vi "Begin.vi"(8 "error in":errorcluster) -> (0 "error out":errorcluster)   [LabVIEW 2023]
doc: "Called before other user functions, this VI is expected to open initial I/O refnums, load in file data, and do all program initialization. Notice that the <B>error out</B> terminal is simply used for data flow. Wiring it to other structures or subVIs ensures that this VI runs first."
uses:
  <vilib>/Rock Robotics/WPI/DriverStation/WPI_DriverStationRobotMode2.ctl
  Robot Global Data.vi
  <vilib>/Rock Robotics/Network Tables/NT Write String Array.vi
  <vilib>/Rock Robotics/WPI/ThirdParty/JAS_Junk/TrajLib/Trajectory_Library.lvlib
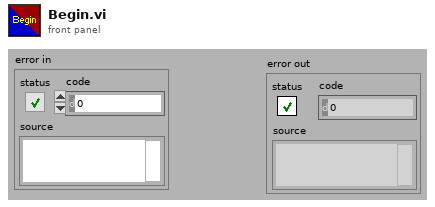
[diagram p1: front panel]
types:
  T1 = cluster{"Future Proof Configs":bool, "MagnetSensorSensorDirection":u16, "MagnetSensorMagnetOffset":dbl, "MagnetSensorAbsoluteSensorDiscontinuityPoint":dbl, "CustomParamsCustomParam0":i16, "CustomParamsCustomParam1":i16}
  T2 = typedef "WPI_DriverStationRobotMode2.ctl" = enum16{"Autonomous Disabled", "Autonomous Enabled", "Teleop Disabled", "Teleop Enabled", "Disconnected", "Finish", "Test Disabled", "Test Enabled", "Emergency Stopped"}
  T3 = typedef "DeviceReference.ctl" = cluster{"CANbus Name":string, "Device Encoding":u32, "Device Name":string}
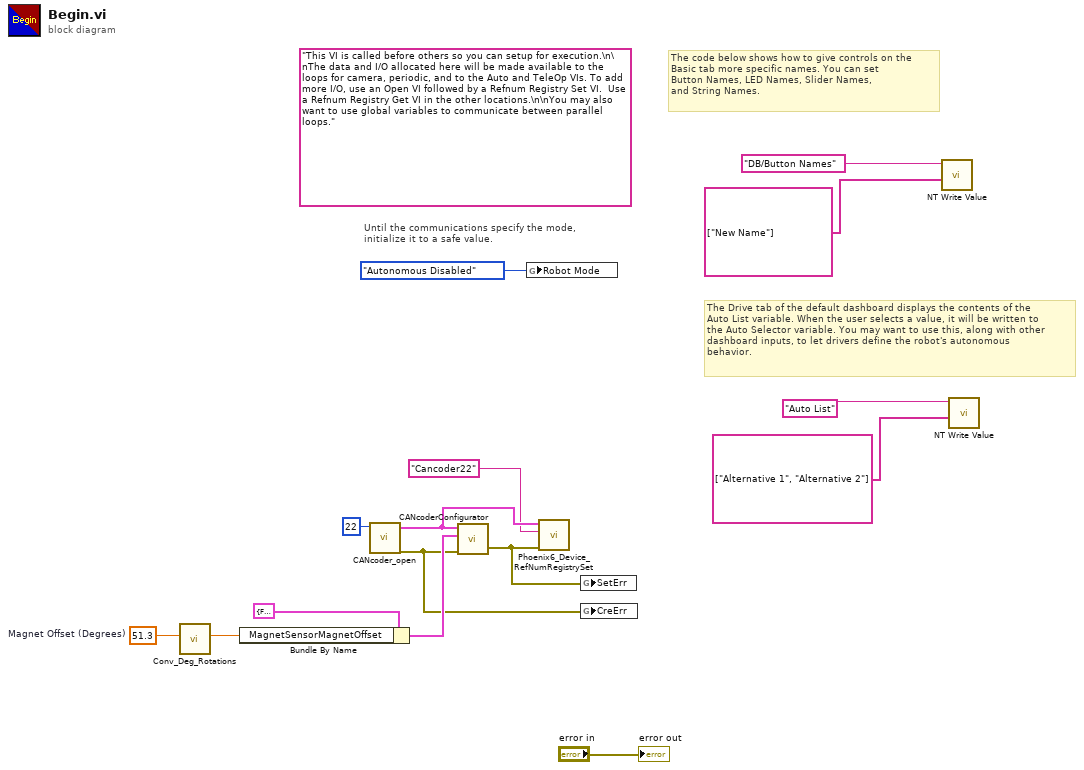
[diagram p0: block diagram]
diagram:
  w4 = 51.3  # Magnet Offset (Degrees)
  (unwired) "This VI is called before others so you can setup for execution.\n\nThe data and I/O allocated here will be made available to the loops for camera, periodic, and to the Auto and TeleOp VIs. To add more I/O, use an Open VI followed by a Refnum Registry Set VI.  Use a Refnum Registry Get VI in the other locations.\n\nYou may also want to use global variables to communicate between parallel loops."
  # "The Drive tab of the default dashboard displays the contents of the\nAuto List variable. When the user selects a value, it will be written to\nthe Auto Selector variable. You may want to use this, along with other\ndashboard inputs, to let drivers define the robot's autonomous\nbehavior."
  # "The code below shows how to give controls on the\nBasic tab more specific names. You can set\nButton Names, LED Names, Slider Names,\nand String Names."
  # "Until the communications specify the mode,\ninitialize it to a safe value."
  n1 = call <vilib>:"Conv_Deg_Rotations.vi"("Degrees"=w4) -> ("Rotations"=w3:dbl)  [unwired: 10 in]
  n2 = Bundle By Name(cluster=T1 {"Future Proof Configs"=FALSE, "MagnetSensorSensorDirection"=0, "MagnetSensorMagnetOffset"=0.0, "MagnetSensorAbsoluteSensorDiscontinuityPoint"=0.5, "CustomParamsCustomParam0"=0, "CustomParamsCustomParam1"=0} ("DeviceConfiguration"), "MagnetSensorMagnetOffset"=w3) -> (w8:T1)
  n3 = call <vilib>:"CANcoder_open.vi"("Device ID"=u8 22) -> ("error out"=w2:errorcluster, "DeviceReference 2"=w7:T3)  [unwired: 9 in]
  n4 = call <vilib>:"CANcoderConfigurator.vi"("error in"=w2, "DeviceConfiguration"=w8, "DeviceReference"=w7) -> ("error out"=w1:errorcluster)  [unwired: 8 in]
  n5 = global write "Robot Global Data.vi" "Robot Mode"(WPI_DriverStationRobotMode2."Autonomous Disabled" ("Robot Mode")) -> ()
  n6 = call <vilib>:"Phoenix6_Device_RefNumRegistrySet.vi"("error in (no error)"=w1, "refnum name"="Cancoder22", "DeviceReference"=w7) -> ()  [unwired: 7 in, 2 out]
  n7 = global write "Robot Global Data.vi" "SetErr"(w1) -> ()
  n8 = global write "Robot Global Data.vi" "CreErr"(w2) -> ()
  n9 = call-poly <vilib>:"NT Write Value.vi"("value"=string[] ["New Name"], "name"="DB/Button Names" ("Name")) -> ()  [unwired: 9 in, 1 out]
  n10 = call-poly <vilib>:"NT Write Value.vi"("value"=string[] ["Alternative 1", "Alternative 2"] ("String Array"), "name"="Auto List" ("Name")) -> ()  [unwired: 9 in, 1 out]
  "error out" <- "error in"
